vi "Reset Supply.vi"(8 "error in":errorcluster, 11 "7976A in":refnum<class "7976A.lvclass">) -> (0 "error out":errorcluster, 3 "7976A out":refnum<class "7976A.lvclass">)   [LabVIEW 2019, in "7976A.lvlib" / "7976A.lvclass"]
uses:
  Library/7976A.lvclass
  C:/Users/Public/Documents/Development/builds/Instruments/PowerSupply.lvlibp/Library/PowerSupply.lvclass
  Library/7976A.lvclass/7976A.ctl
  builds/Instruments/PowerSupply.lvlibp/Library/PowerSupply.lvclass
  <instrlib>/Agilent N7976A/Agilent N7976A.lvlib
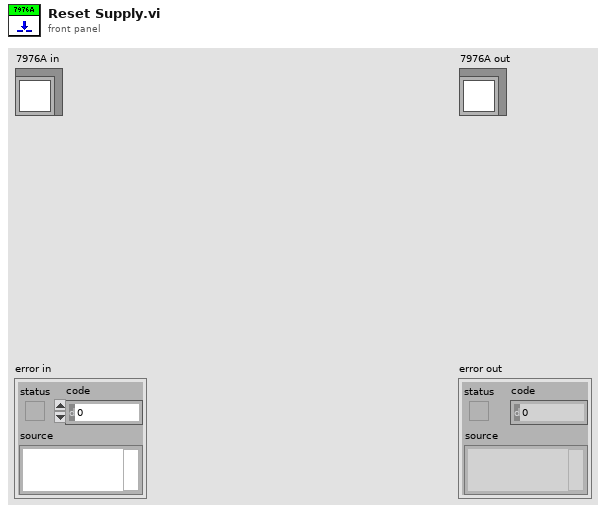
[diagram p1: front panel]
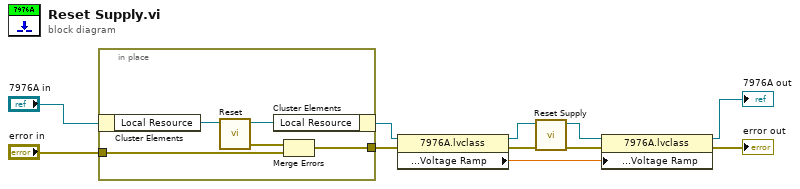
[diagram p0: block diagram]
diagram:
  n1 = in-place {
    in-place-border: "error in" -> [w13]
    in-place-border: [w12] -> w8
    n2 = in-place-cluster #1("7976A in") -> ("Local Resource"=w16:refnum<visa-resource-name>)
    n3 = call <instrlib>:"Reset.vi"("VISA resource name"=w16) -> ("error out"=w14:errorcluster, "VISA resource name out"=w15:refnum<visa-resource-name>)  [unwired: 9 in]
    n4 = in-place-cluster #1("Local Resource"=w15) -> (w6:refnum<class "7976A.lvclass">)
    n5 = Merge Errors(w14, w13) -> (w12:errorcluster)
  }
  n6 = property class="7976A.lvclass"(reference=w6, error in=w8) -> (reference out=w5:refnum<class "7976A.lvclass">, error out=w7:errorcluster, "Accessors:Setting:Ramp:Voltage Ramp"=w1:dbl)
  n7 = call-parent "Reset Supply.vi"("error in"=w7, "PowerSupply in"=w5) -> ("error out"=w11:errorcluster, "PowerSupply out"=w3:refnum<class "7976A.lvclass">)  [unwired: 8 in]
  n8 = property class="7976A.lvclass"(reference=w3, error in=w11, "Accessors:Setting:Ramp:Voltage Ramp"=w1) -> (reference out=→"7976A out":refnum<class "7976A.lvclass">, error out=→"error out":errorcluster)
